vi "hex to binary.vi"(11 "字符串":string) -> (0 "Result":string, 3 "二进制":string)   [LabVIEW 2013]
panel:
  out "二进制数值":u32 format="%08b"
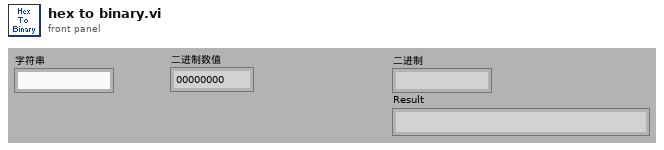
[diagram p1: front panel]
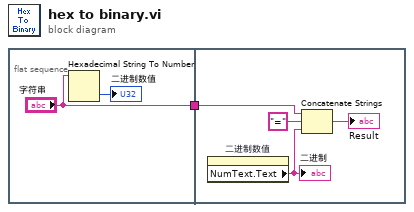
[diagram p0: block diagram]
diagram:
  n1 = flat-sequence {
    tunnel: ["字符串"] -> w1
    tunnel: w1 -> [w7]
    frame #0 {
      n2 = Hexadecimal String To Number(string="字符串") -> (number=→"二进制数值":u32)  [unwired: 2 in, 1 out]
    }
    frame #1 {
      n3 = property on="二进制数值" class="DigNum (strict)"() -> ("NumText.Text"=w5:string)  [unwired: 2 in, 2 out]
      "二进制" <- w5
      n4 = Concatenate Strings(w7, "=" ("字符串"), w5) -> (→"Result":string)
    }
  }
